vi "Test - Copy State From CSM to CSM.vi"() -> ()   [LabVIEW 2020]
uses:
  _csmHelper/API/Create From VI Reference.vi
  _csmHelper/API/Open Block Diagram.vi
  _csmHelper/API/Destroy.vi
  _csmHelper/API/Stop Undo.vi
  _csmHelper/API/Copy State.vi
  _csmHelper/API/Start Undo.vi
  _csmHelper/CSM-Helper.lvclass
panel:
  in  "State":string="Error Handler"
  # "Error Handler"
  # "Data: Initialize"
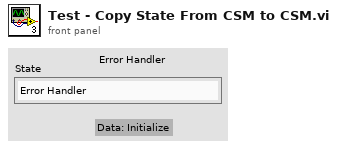
[diagram p1: front panel]
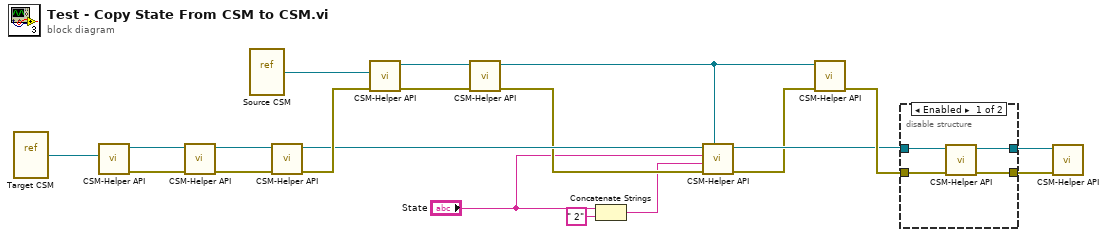
[diagram p0: block diagram]
diagram:
  n1 = vi-ref "Target CSM.vi"() -> (w19:refnum<vi>)
  n2 = call-poly "CSM-Helper API.vi"("VI"=w19) -> ("error out"=w11:errorcluster, "CSM-Helper.lvclass"=w10:refnum<class "CSM-Helper.lvclass">)  [unwired: 9 in]
  n3 = call-poly "CSM-Helper API.vi"("error in (no error)"=w11, "CSM-Helper in"=w10) -> ("error out"=w9:errorcluster, "CSM-Helper out"=w8:refnum<class "CSM-Helper.lvclass">)  [unwired: 8 in]
  n4 = vi-ref "Source CSM.vi"() -> (w20:refnum<vi>)
  n5 = call-poly "CSM-Helper API.vi"("error in (no error)"=w9, "CSM-Helper in"=w8) -> ("error out"=w13:errorcluster, "CSM-Helper out"=w12:refnum<class "CSM-Helper.lvclass">)  [unwired: 8 in]
  n6 = call-poly "CSM-Helper API.vi"("error in (no error)"=w13, "VI"=w20) -> ("error out"=w5:errorcluster, "CSM-Helper.lvclass"=w7:refnum<class "CSM-Helper.lvclass">)  [unwired: 8 in]
  n7 = call-poly "CSM-Helper API.vi"("error in (no error)"=w5, "CSM-Helper in"=w7) -> ("error out"=w4:errorcluster, "CSM-Helper out"=w6:refnum<class "CSM-Helper.lvclass">)  [unwired: 8 in]
  n8 = Concatenate Strings("State", " 2" ("string")) -> (w2:string)
  n9 = call-poly "CSM-Helper API.vi"("SourceCSM"=w6, "error in (no error)"=w4, "New(Empty to Use same Name)"=w2, "Case"="State", "CSM-Helper.lvclass"=w12) -> ("error out"=w14:errorcluster, "CSM-Helper out 2"=w15:refnum<class "CSM-Helper.lvclass">)  [unwired: 5 in]
  n10 = call-poly "CSM-Helper API.vi"("error in (no error)"=w14, "CSM-Helper in"=w6) -> ("error out"=w17:errorcluster)  [unwired: 8 in, 1 out]
  n11 = disable-structure shown="Enabled" {
    disable-tunnel: [w24 w26] -> w18
    disable-tunnel: w17 -> [w23 w25]
    disable-tunnel: [w22 w25] -> w16
    disable-tunnel: w15 -> [w21 w26]
    frame Enabled {
      n12 = call-poly "CSM-Helper API.vi"("error in (no error)"=w23, "CSM-Helper in"=w21) -> ("error out"=w22:errorcluster, "CSM-Helper out"=w24:refnum<class "CSM-Helper.lvclass">)  [unwired: 8 in]
    }
    frame Disabled {
    }
  }
  n13 = call-poly "CSM-Helper API.vi"("error in (no error)"=w16, "CSM-Helper in"=w18) -> ()  [unwired: 8 in, 2 out]
